vi "状态匹配.vi"(11 "输入状态":string) -> (3 "输出状态":string)   [LabVIEW 2018]
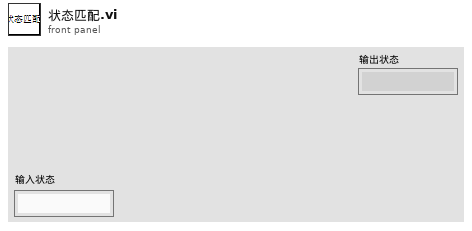
[diagram p1: front panel]
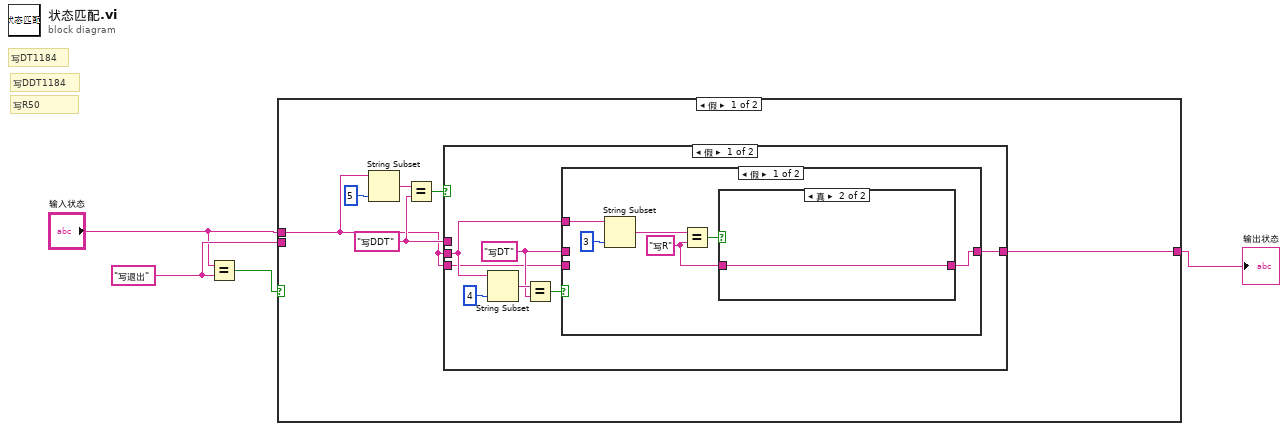
[diagram p0: block diagram]
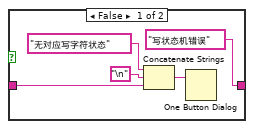
[diagram p2: hidden frame]
diagram:
  w4 = "写退出" ("y")
  # "写R50"
  # "写DDT1184"
  # "写DT1184"
  n1 = Equal?(x="输入状态", y=w4) -> (x = y?=w1:bool)
  n2 = case shown="假" w1 {
    tunnel: "输入状态" -> [w6 _]
    tunnel: [w5 w32] -> w3
    tunnel: w4 -> [_ w32]
    frame False {
      w7 = "写DDT" ("y")
      n3 = String Subset(string=w6, length (rest)=5 ("长度（剩余）")) -> (substring=w9:string)  [unwired: 1 in]
      n4 = Equal?(x=w9, y=w7) -> (x = y?=w8:bool)
      n5 = case shown="假" w8 {
        tunnel: w6 -> [w13 _]
        tunnel: [w11 w31] -> w5
        tunnel: w7 -> [_ w31]
        tunnel: w6 -> [w12 _]
        frame False {
          w14 = "写DT" ("y")
          n6 = String Subset(string=w13, length (rest)=4 ("长度（剩余）")) -> (substring=w16:string)  [unwired: 1 in]
          n7 = Equal?(x=w16, y=w14) -> (x = y?=w15:bool)
          n8 = case shown="假" w15 {
            tunnel: w14 -> [_ w30]
            tunnel: [w19 w30] -> w11
            tunnel: w13 -> [w23 _]
            tunnel: w12 -> [_ _]
            frame False {
              w18 = "写R" ("y")
              n9 = String Subset(string=w23, length (rest)=3 ("长度（剩余）")) -> (substring=w21:string)  [unwired: 1 in]
              n10 = Equal?(x=w21, y=w18) -> (x = y?=w20:bool)
              n11 = case shown="真" w20 {
                tunnel: w18 -> [w25 w29]
                tunnel: ["写状态机错误" ("字符串") w29] -> w19
                frame False {
                  n12 = Concatenate Strings("无对应写字符状态" ("字符串"), "\n", w25) -> (w27:string)
                  n13 = One Button Dialog(message=w27) -> ()  [unwired: 1 in, 1 out]
                }
                frame True {
                }
              }
            }
            frame True {
            }
          }
        }
        frame True {
        }
      }
    }
    frame True {
    }
  }
  "输出状态" <- w3
